vi "Tuncate_Cluster.vi"(10 "Eingangscluster":T1) -> (2 "Cluster":T1)   [LabVIEW 2016]
uses:
  Instrument_Setup.vi
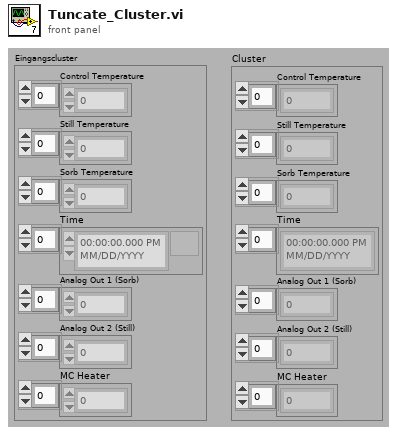
[diagram p1: front panel]
types:
  T1 = cluster{"Control Temperature":dbl[], "Still Temperature":dbl[], "Sorb Temperature":dbl[], "Time":timestamp[], "Analog Out 1 (Sorb)":dbl[], "Analog Out 2 (Still)":dbl[], "MC Heater":dbl[]}
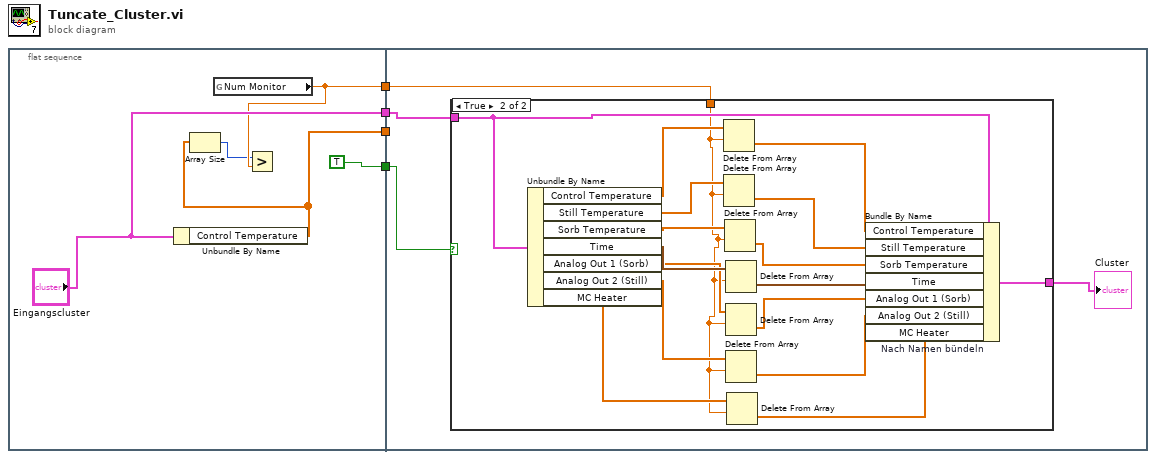
[diagram p0: block diagram]
diagram:
  n1 = flat-sequence {
    tunnel: [w6] -> w4
    tunnel: ["Eingangscluster"] -> w3
    tunnel: [w8] -> w2
    tunnel: [TRUE] -> w1
    tunnel: w4 -> [_]
    tunnel: w3 -> [w13]
    tunnel: w2 -> [w10]
    tunnel: w1 -> [w12]
    frame #0 {
      n2 = Unbundle By Name("Eingangscluster") -> ("Control Temperature"=w6:dbl[])
      n3 = Array Size(array=w6) -> (size(s)=w7:i32)
      n4 = global read "Instrument_Setup.vi" "Num Monitor"() -> (w8:dbl)
      n5 = Greater?(x=w7, y=w8) -> ()  [unwired: 1 out]
    }
    frame #1 {
      n6 = case shown="True" w12 {
        tunnel: w13 -> [w14 w24]
        tunnel: w10 -> [_ w16]
        tunnel: [w14 w15] -> w11
        frame False {
        }
        frame True {
          n7 = Unbundle By Name(w24) -> ("Control Temperature"=w23:dbl[], "Still Temperature"=w22:dbl[], "Sorb Temperature"=w21:dbl[], "Time"=w20:timestamp[], "Analog Out 1 (Sorb)"=w19:dbl[], "Analog Out 2 (Still)"=w18:dbl[], "MC Heater"=w17:dbl[])
          n8 = Delete From Array(array=w23, length=w16) -> (deleted portion=w31:dbl[])  [unwired: 1 in, 1 out]
          n9 = Delete From Array(array=w22, length=w16) -> (deleted portion=w30:dbl[])  [unwired: 1 in, 1 out]
          n10 = Delete From Array(array=w21, length=w16) -> (deleted portion=w29:dbl[])  [unwired: 1 in, 1 out]
          n11 = Delete From Array(array=w20, length=w16) -> (deleted portion=w28:timestamp[])  [unwired: 1 in, 1 out]
          n12 = Delete From Array(array=w19, length=w16) -> (deleted portion=w27:dbl[])  [unwired: 1 in, 1 out]
          n13 = Delete From Array(array=w18, length=w16) -> (deleted portion=w26:dbl[])  [unwired: 1 in, 1 out]
          n14 = Delete From Array(array=w17, length=w16) -> (deleted portion=w25:dbl[])  [unwired: 1 in, 1 out]
          n15 = Bundle By Name "Nach Namen bündeln"(cluster=w24, "Control Temperature"=w31, "Still Temperature"=w30, "Sorb Temperature"=w29, "Time"=w28, "Analog Out 1 (Sorb)"=w27, "Analog Out 2 (Still)"=w26, "MC Heater"=w25) -> (w15:T1)
        }
      }
      "Cluster" <- w11
    }
  }
